vi "get_source_parameters_cluster.vi"(8 "error in (no error)":errorcluster, 10 "Source number":u8, 11 "VISA resource name":refnum<visa-resource-name>) -> (0 "error out":errorcluster, 2 "Source parameters":T1, 3 "VISA resource name out":refnum<visa-resource-name>)   [LabVIEW 2018]
doc: "Set the density of a material."
uses:
  Low Level/source_parameter_ring.ctl
  Low Level/source_parameters_strings.ctl
  Low Level/source_parameters.ctl
panel:
  in  "Source parameters (strings)":T2
  in  "Source parameter":T3 items=["DAC Output", "Shutter Output", "Number of Crucibles", "Crucible Output", "Turret Feedback", "Turret Input", "Turret Delay (s)"]
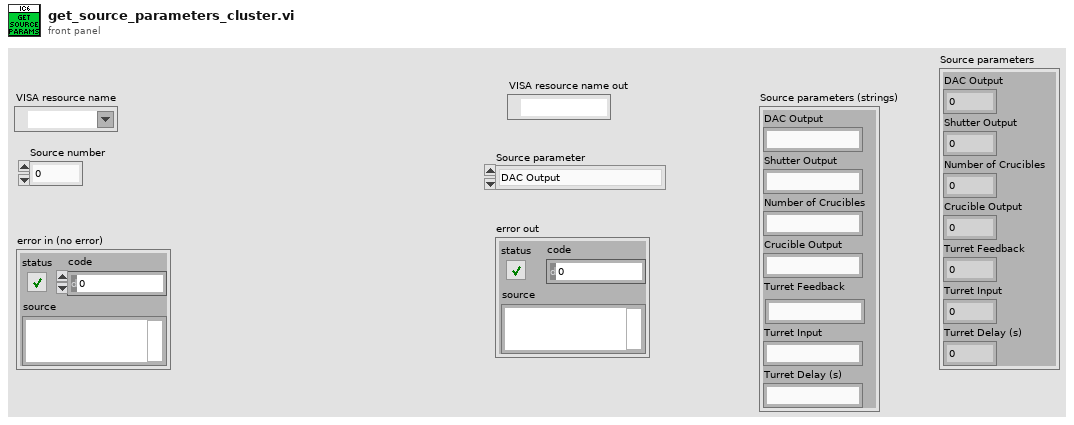
[diagram p1: front panel]
types:
  T1 = typedef "source_parameters.ctl" = cluster{"DAC Output":u8, "Shutter Output":u8, "Number of Crucibles":u8, "Crucible Output":u8, "Turret Feedback":u8, "Turret Input":u8, "Turret Delay (s)":u8}
  T2 = typedef "source_parameters_strings.ctl" = cluster{"DAC Output":string, "Shutter Output":string, "Number of Crucibles":string, "Crucible Output":string, "Turret Feedback":string, "Turret Input":string, "Turret Delay (s)":string}
  T3 = typedef "source_parameter_ring.ctl" = u16
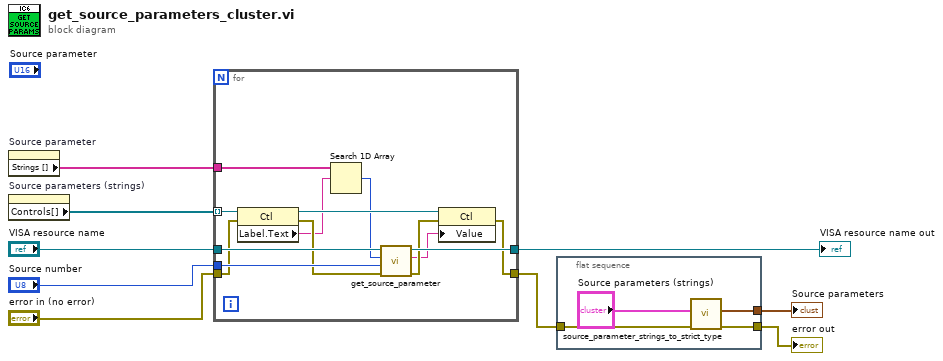
[diagram p0: block diagram]
diagram:
  n1 = property on="Source parameter" class="Ring (strict)"() -> ("Strings []"=w5:string[])  [unwired: 2 in, 2 out]
  n2 = property on="Source parameters (strings)" class="Clust (strict)"() -> ("Controls[]"=w1:refnum<vi>[])  [unwired: 2 in, 2 out]
  n3 = for {
    tunnel: "VISA resource name" -> [w22]
    tunnel: [w21] -> w8
    tunnel: [w13] -> w3
    tunnel: "error in (no error)" -> [w17]
    tunnel: "Source number" -> [w20]
    tunnel: w5 -> [w19]
    tunnel: w1 -> [w18] mode=indexing
    n4 = property class="Ctl"(reference=w18, error in=w17) -> (reference out=w15:refnum<vi>, error out=w16:errorcluster, "Label.Text"=w12:string)
    n5 = Search 1D Array(1D array=w19, element=w12) -> (index of element=w10:i32)  [unwired: 1 in]
    n6 = call "get_source_parameter.vi"("error in (no error)"=w16, "Source number"=w20, "Source parameter"=w10, "VISA resource name"=w22) -> ("error out"=w14:errorcluster, "Source parameter value"=w11:string, "VISA resource name out"=w21:refnum<visa-resource-name>)  [unwired: 5 in]
    n7 = property class="Ctl"(reference=w15, error in=w14, "Value"=w11) -> (error out=w13:errorcluster)  [unwired: 1 out]
  }
  "VISA resource name out" <- w8
  n8 = flat-sequence {
    tunnel: [w24] -> w4
    tunnel: w3 -> [w25]
    tunnel: [w23] -> w2
    frame #0 {
      n9 = call "source_parameter_strings_to_strict_type.vi"("error in (no error)"=w25, "Source parameters (strings)"="Source parameters (strings)") -> ("error out"=w24:errorcluster, "Source parameters"=w23:T1)  [unwired: 8 in]
    }
  }
  "error out" <- w4
  "Source parameters" <- w2
